vi "Excel_Format.vi"(8 "error in (no error)":errorcluster, 9 "Backup path":path, 10 "file path":path) -> (0 "error out":errorcluster)   [LabVIEW 2015]
doc: "格式化报表的字体"
uses:
  <vilib>/Utility/NIReport.llb/NI_report.lvclass
  <vilib>/Utility/NIReport.llb/Excel/NI_Excel.lvclass
panel:
  in  "start(-1,-1)":cluster{"row":i32, "column":i32}
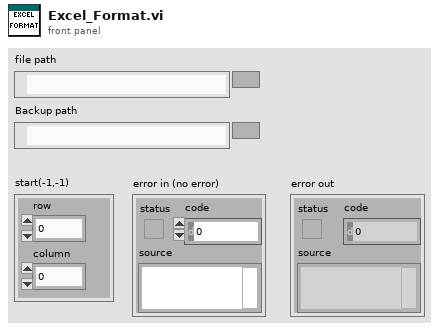
[diagram p1: front panel]
types:
  T1 = enum16{"Standard Report", "HTML", "Word", "Excel"}
  T2 = enum16{"maximized", "minimized", "normal", "no change"}
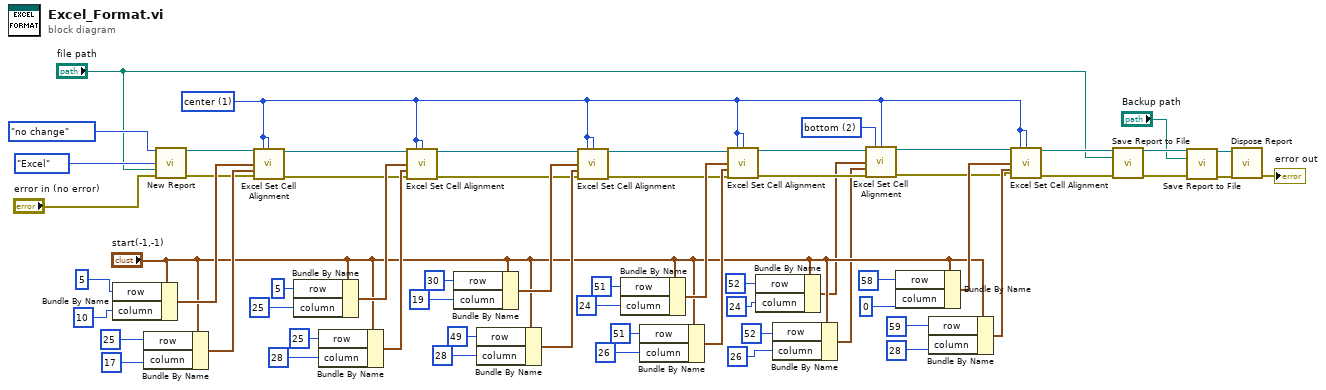
[diagram p0: block diagram]
diagram:
  w12 = 2 items=["top", "center", "bottom"] ("vertical alignment (top)")
  w11 = 1 items=["top", "center", "bottom"] ("vertical alignment (top)")
  n1 = Bundle By Name(cluster="start(-1,-1)", "row"=5, "column"=10) -> (w63:cluster{"row":i32, "column":i32})
  n2 = Bundle By Name(cluster="start(-1,-1)", "row"=25 ("column"), "column"=17) -> (w62:cluster{"row":i32, "column":i32})
  n3 = call <vilib>:"New Report.vi"("window state (normal)"=T2."no change", "report type"=T1."Excel", "template (empty)"="file path", "error in (no error)"="error in (no error)") -> ("report out"=w45:refnum<class "NI_report.lvclass">, "error out"=w43:errorcluster)  [unwired: 10 in]
  n4 = call <vilib>:"Excel Set Cell Alignment.vi"("report in"=w45, "vertical alignment (top)"=w11, "horizontal alignment (left)"=w11, "start (-1, -1)"=w63, "end (-1, -1)"=w62, "error in (no error)"=w43) -> ("report out"=w44:refnum<class "NI_report.lvclass">, "error out"=w42:errorcluster)  [unwired: 8 in]
  n5 = Bundle By Name(cluster="start(-1,-1)", "row"=5, "column"=25) -> (w55:cluster{"row":i32, "column":i32})
  n6 = Bundle By Name(cluster="start(-1,-1)", "row"=25, "column"=28) -> (w54:cluster{"row":i32, "column":i32})
  n7 = call <vilib>:"Excel Set Cell Alignment.vi"("report in"=w44, "vertical alignment (top)"=w11, "horizontal alignment (left)"=w11, "start (-1, -1)"=w55, "end (-1, -1)"=w54, "error in (no error)"=w42) -> ("report out"=w40:refnum<class "NI_report.lvclass">, "error out"=w41:errorcluster)  [unwired: 8 in]
  n8 = Bundle By Name(cluster="start(-1,-1)", "row"=30, "column"=19) -> (w51:cluster{"row":i32, "column":i32})
  n9 = Bundle By Name(cluster="start(-1,-1)", "row"=49, "column"=28) -> (w50:cluster{"row":i32, "column":i32})
  n10 = call <vilib>:"Excel Set Cell Alignment.vi"("report in"=w40, "vertical alignment (top)"=w11, "horizontal alignment (left)"=w11, "start (-1, -1)"=w51, "end (-1, -1)"=w50, "error in (no error)"=w41) -> ("report out"=w33:refnum<class "NI_report.lvclass">, "error out"=w32:errorcluster)  [unwired: 8 in]
  n11 = Bundle By Name(cluster="start(-1,-1)", "row"=51, "column"=24) -> (w39:cluster{"row":i32, "column":i32})
  n12 = Bundle By Name(cluster="start(-1,-1)", "row"=51, "column"=26) -> (w38:cluster{"row":i32, "column":i32})
  n13 = call <vilib>:"Excel Set Cell Alignment.vi"("report in"=w33, "vertical alignment (top)"=w11, "horizontal alignment (left)"=w11, "start (-1, -1)"=w39, "end (-1, -1)"=w38, "error in (no error)"=w32) -> ("report out"=w18:refnum<class "NI_report.lvclass">, "error out"=w17:errorcluster)  [unwired: 8 in]
  n14 = Bundle By Name(cluster="start(-1,-1)", "row"=52, "column"=24) -> (w14:cluster{"row":i32, "column":i32})
  n15 = Bundle By Name(cluster="start(-1,-1)", "row"=52, "column"=26) -> (w13:cluster{"row":i32, "column":i32})
  n16 = call <vilib>:"Excel Set Cell Alignment.vi"("report in"=w18, "vertical alignment (top)"=w12, "horizontal alignment (left)"=w11, "start (-1, -1)"=w14, "end (-1, -1)"=w13, "error in (no error)"=w17) -> ("report out"=w16:refnum<class "NI_report.lvclass">, "error out"=w15:errorcluster)  [unwired: 8 in]
  n17 = Bundle By Name(cluster="start(-1,-1)", "row"=58, "column"=0) -> (w31:cluster{"row":i32, "column":i32})
  n18 = Bundle By Name(cluster="start(-1,-1)", "row"=59, "column"=28) -> (w30:cluster{"row":i32, "column":i32})
  n19 = call <vilib>:"Excel Set Cell Alignment.vi"("report in"=w16, "vertical alignment (top)"=w11, "horizontal alignment (left)"=w11, "start (-1, -1)"=w31, "end (-1, -1)"=w30, "error in (no error)"=w15) -> ("report out"=w29:refnum<class "NI_report.lvclass">, "error out"=w28:errorcluster)  [unwired: 8 in]
  n20 = call-dynamic "Save Report to File.vi"("report in"=w29, "report file path"="file path", "error in (no error)"=w28) -> ("report out"=w6:refnum<class "NI_report.lvclass">, "error out"=w5:errorcluster)  [unwired: 11 in]
  n21 = call-dynamic "Save Report to File.vi"("report in"=w6, "report file path"="Backup path", "error in (no error)"=w5) -> ("report out"=w4:refnum<class "NI_report.lvclass">, "error out"=w3:errorcluster)  [unwired: 11 in]
  n22 = call-dynamic "Dispose Report.vi"("report in"=w4, "error in (no error)"=w3) -> ("error out"=→"error out":errorcluster)  [unwired: 13 in]
